vi "startUI.vi"(8 "error in (no error)":errorcluster, 10 "AMC*":T1, 11 "Channel in":refnum<class "Parameter.lvclass">) -> (0 "error out":errorcluster, 2 "UI VI*":refnum<vi>, 3 "Channel out":refnum<class "Parameter.lvclass">)   [LabVIEW 2013, in "Parameter.lvclass"]
doc: "Starts the user interface VI for this xceDataNode. This is the precursor to loading the UI VI into the xceSubpanel class. Also this VI is dynamic dispatch because it is just the suggested way to start a dynamic VI. This has been created with the idea that your classes UI VI will be created from the DataNodeUI.vit template."
uses:
  Parameter.lvclass
  <vilib>/NI/AMC/Message Queue.ctl
  <vilib>/NI/AMC/Message.ctl
  <vilib>/NI/Tools/Keyed Array/KeyedArray.ctl
  xCE/xceNode/xceNode.lvclass
  xCE/xceDataNode/xceDataNode.lvclass
  <vilib>/NI/AMC/AMC.lvlib
  <vilib>/NI/Tools/Keyed Array/Tools_KeyedArray.lvlib
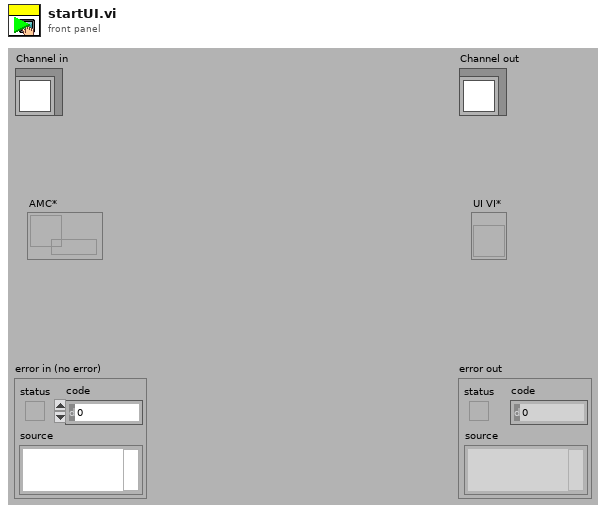
[diagram p1: front panel]
types:
  T1 = typedef "AMC.lvlib/Message Queue.ctl" = refnum<queue>
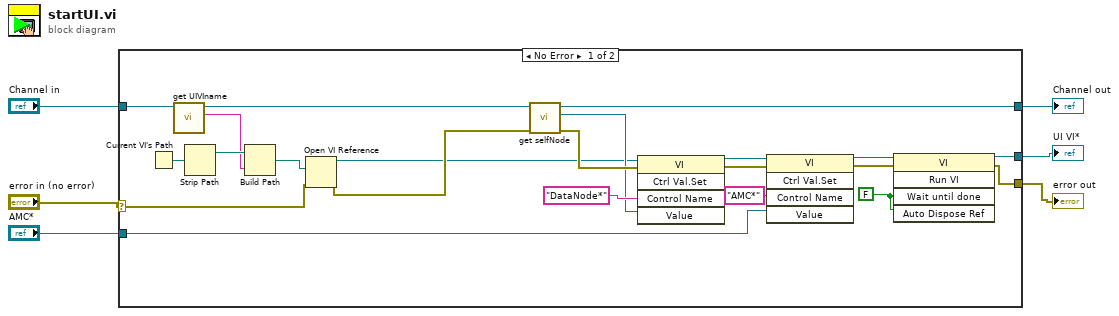
[diagram p0: block diagram]
diagram:
  n1 = case shown="No Error" "error in (no error)" {
    selector: "error in (no error)" -> [w11 w30]
    tunnel: [w19 w30] -> w1
    tunnel: [w27 w29] -> w3
    tunnel: "Channel in" -> [w12 w29]
    tunnel: "AMC*" -> [w23 _]
    tunnel: [w18 _] -> w2
    frame No Error {
      w20 = FALSE ("Wait Until Done")
      n2 = Current VI's Path() -> (path=w14:path)
      n3 = call "get UIVIname.vi"("xceDataNode in"=w12) -> ("UI VI name"=w8:string, "xceDataNode out"=w9:refnum<class "Parameter.lvclass">)  [unwired: 8 in, 1 out]
      n4 = Strip Path(path=w14) -> (stripped path=w13:path)  [unwired: 1 out]
      n5 = Build Path(base path=w13, name or relative path=w8) -> (appended path=w15:path)
      n6 = Open VI Reference(vi path=w15, error in (no error)=w11) -> (vi reference=w7:refnum<vi>, error out=w10:errorcluster)  [unwired: 4 in]
      n7 = call "get selfNode.vi"("error in (no error)"=w10, "xceNode in"=w9) -> ("error out"=w17:errorcluster, "selfNode*"=w16:refnum<data-value>, "xceNode out"=w27:refnum<class "Parameter.lvclass">)  [unwired: 7 in]
      n8 = invoke class="VI" method="Ctrl Val.Set"(reference=w7, error in=w17, "Control Name"="DataNode*", "Value"=w16) -> (reference out=w26:refnum<vi>, error out=w25:errorcluster)  [unwired: 1 in, 3 out]
      n9 = invoke class="VI" method="Ctrl Val.Set"(reference=w26, error in=w25, "Control Name"="AMC*", "Value"=w23) -> (reference out=w22:refnum<vi>, error out=w21:errorcluster)  [unwired: 1 in, 3 out]
      n10 = invoke class="VI" method="Run VI"(reference=w22, error in=w21, "Wait until done"=w20, "Auto Dispose Ref"=w20) -> (reference out=w18:refnum<vi>, error out=w19:errorcluster)  [unwired: 1 in, 3 out]
    }
    frame Error {
    }
  }
  "error out" <- w1
  "Channel out" <- w3
  "UI VI*" <- w2
